vi "neuron.vi"(4 "weight 3":fxp<+/-,64,32>, 6 "input 3":fxp<+/-,64,32>, 7 "input 1":fxp<+/-,64,32>, 9 "weight 2":fxp<+/-,64,32>, 10 "input 2":fxp<+/-,64,32>, 11 "weight 1":fxp<+/-,64,32>) -> (3 "activation":fxp<+/-,64,32>)   [LabVIEW 2015]
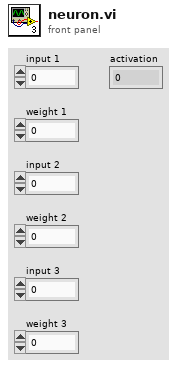
[diagram p1: front panel]
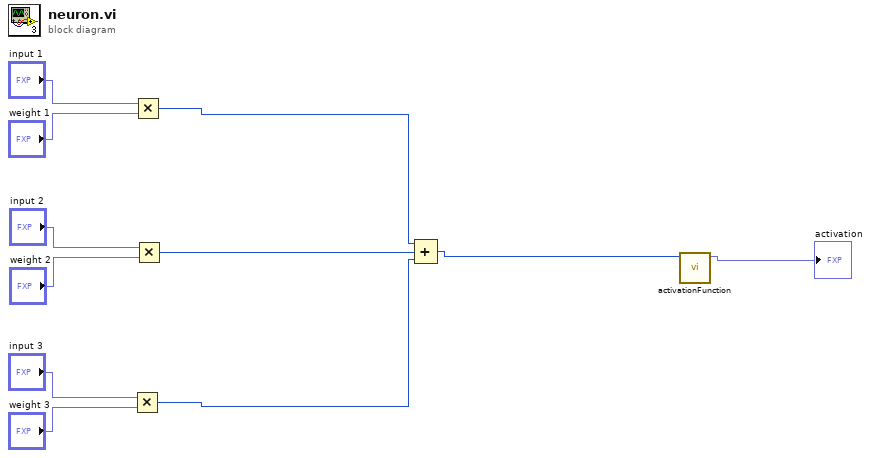
[diagram p0: block diagram]
diagram:
  n1 = Multiply(x="input 3", y="weight 3") -> (x*y=w2:i16)
  n2 = Multiply(x="input 1", y="weight 1") -> (x*y=w4:i16)
  n3 = Multiply(x="input 2", y="weight 2") -> (x*y=w3:i16)
  n4 = Compound Arithmetic op=ADD(w4, w3, w2) -> (w1:i16)
  n5 = call "activationFunction.vi"("input"=w1) -> ("activation"=→"activation":fxp<+/-,64,32>)  [unwired: 10 in]
